vi "Create Sections Headings.vi"(11 "sections":string[](array[string])) -> (0 "sections end":string, 2 "spaces number":i32, 3 "sections start":string)   [LabVIEW 2013, in "infolib.lvlib"]
doc: "Creates headings and tails for structure of sections. Returns also appropriate number of indent spaces for the sections content."
uses:
  infolib.lvlib
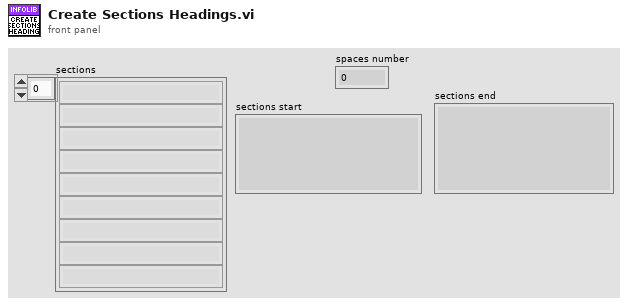
[diagram p1: front panel]
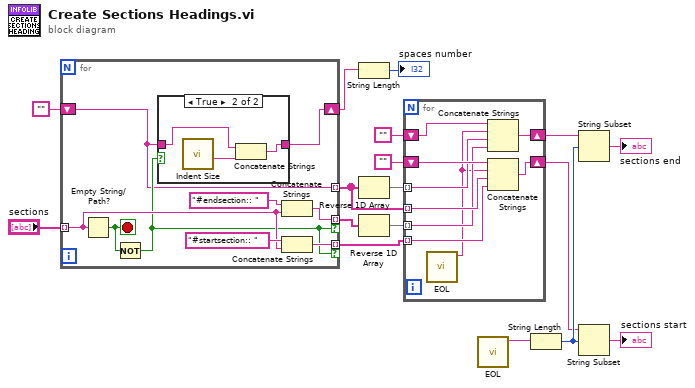
[diagram p0: block diagram]
diagram:
  n1 = for {
    tunnel: "sections" -> [w22] mode=indexing
    shift-right: [w25] -> w2
    shift-left: "" -> [w18]
    tunnel: [w18] -> w10 mode=indexing
    tunnel: [w21] -> w12 mode=indexing if=w19
    tunnel: [w20] -> w5 mode=indexing if=w19
    stop <- w26 stop-if-true
    n2 = Empty String/Path?(string/path=w22) -> (empty?=w26:bool)
    n3 = Not(x=w26) -> (.not. x?=w19:bool)
    n4 = case shown="True" w19 {
      tunnel: w18 -> [w27 w30]
      tunnel: [w27 w29] -> w25
      frame False {
      }
      frame True {
        n5 = call "Indent Size.vi"() -> ("indent"=w28:string)  [unwired: 10 in, 1 out]
        n6 = Concatenate Strings(w30, w28) -> (w29:string)
      }
    }
    n7 = Concatenate Strings("#endsection:: " ("string"), w22) -> (w20:string)
    n8 = Concatenate Strings("#startsection:: " ("string"), w22) -> (w21:string)
  }
  n9 = String Length(string=w2) -> (length=→"spaces number":i32)
  n10 = Reverse 1D Array(array=w10) -> (reversed array=w9:string[])
  n11 = Reverse 1D Array(array=w5) -> (reversed array=w4:string[])
  n12 = for {
    tunnel: w12 -> [w34] mode=indexing
    tunnel: w10 -> [w35] mode=indexing
    shift-right: [w38] -> w6
    shift-left: "" -> [w39]
    tunnel: w9 -> [w32] mode=indexing
    shift-right: [w36] -> w7
    shift-left: "" -> [w37]
    tunnel: w4 -> [w33] mode=indexing
    n13 = call "EOL.vi"() -> ("eol"=w31:string)  [unwired: 11 in]
    n14 = Concatenate Strings(w37, w31, w32, w33) -> (w36:string)
    n15 = Concatenate Strings(w39, w31, w35, w34) -> (w38:string)
  }
  n16 = call "EOL.vi"() -> ("eol"=w3:string)  [unwired: 11 in]
  n17 = String Length(string=w3) -> (length=w13:i32)
  n18 = String Subset(string=w7, offset (0)=w13) -> (substring=→"sections end":string)  [unwired: 1 in]
  n19 = String Subset(string=w6, offset (0)=w13) -> (substring=→"sections start":string)  [unwired: 1 in]
